vi "Main.vi"(8 "error in (no error)":errorcluster, 11 "Stop notifier":refnum<notifier>) -> (0 "error out":errorcluster)   [LabVIEW 2017, in "Temp.lvlib"]
doc: "Module main"
uses:
  Temp.lvlib
  ctl/StateData.ctl
  ctl/MainStates.ctl
  <vilib>/ErrorRing/Error Ring.xnode
  Error/Error.lvlib
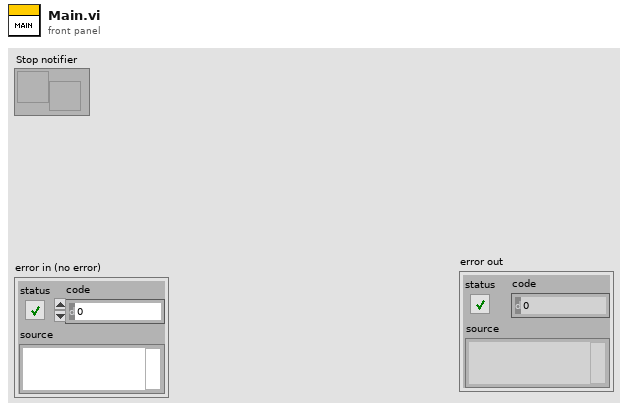
[diagram p1: front panel]
types:
  T1 = typedef "Temp.lvlib/StateData.ctl" = cluster{"Blank":dbl}
  T2 = typedef "Temp.lvlib/MainStates.ctl" = enum16{"Timeout", "Error", "Exit", "Init"}
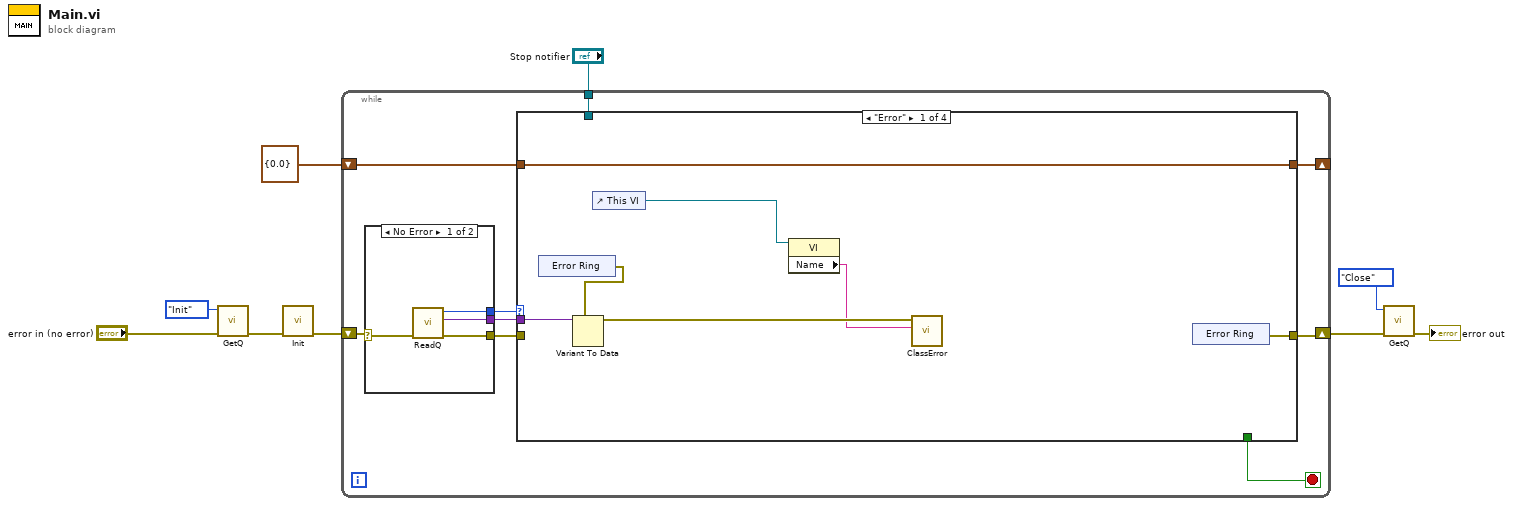
[diagram p0: block diagram]
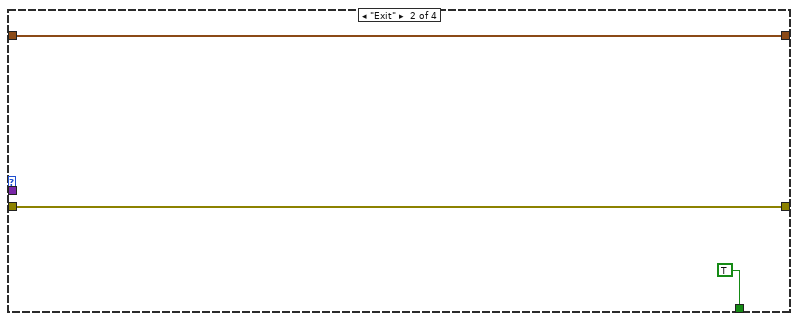
[diagram p2: hidden frame]
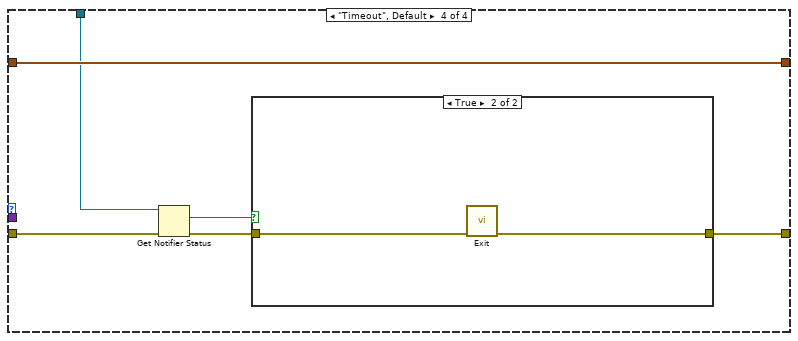
[diagram p4: hidden frame]
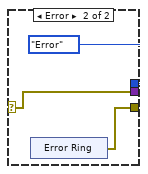
[diagram p6: hidden frame]
diagram:
  n1 = call "GetQ.vi"("error in (no error)"="error in (no error)", "Mode (Get)"=enum16{"Get", "Close", "Init"}."Init") -> ("error out"=w2:errorcluster)  [unwired: 8 in, 1 out]
  n2 = call "Init.vi"("error in (no error)"=w2) -> ("error out"=w1:errorcluster)  [unwired: 10 in]
  n3 = while {
    shift-right: [w14] -> w6
    shift-left: w1 -> [w18]
    shift-right: [w11] -> _
    shift-left: T1 {"Blank"=0.0} ("Cluster") -> [w12]
    tunnel: "Stop notifier" -> [w10]
    stop <- w13 stop-if-true
    n4 = case shown="No Error" w18 {
      selector: w18 -> [w45 w47]
      tunnel: [w44 MainStates."Error" ("State")] -> w17
      tunnel: [w43 w47] -> w16
      tunnel: [w42 w46] -> w15
      frame No Error {
        n5 = call "ReadQ.vi"("error in (no error)"=w45) -> ("error out"=w42:errorcluster, "Variant"=w43:variant, "State"=w44:T2)  [unwired: 8 in]
      }
      frame Error {
        n6 = xnode "Error Ring"() -> ("error out"=w46:errorcluster)
      }
    }
    n7 = case shown="\"Error\"" w17 {
      tunnel: w16 -> [w25 _ _ _]
      tunnel: w15 -> [_ w30 w32 w37]
      tunnel: [w24 w30 w32 w34] -> w14
      tunnel: [_ TRUE _ _] -> w13
      tunnel: w12 -> [w22 w28 w31 w38]
      tunnel: [w22 w28 w31 w38] -> w11
      tunnel: w10 -> [_ _ _ w36]
      frame "Error" {
        n8 = xnode "Error Ring"() -> ("error out"=w23:errorcluster)
        n9 = Variant To Data(type=w23, Variant=w25) -> (data=w21:errorcluster)  [unwired: 1 in, 1 out]
        n10 = control-ref of="This VI"() -> (w20:refnum<vi>)
        n11 = property class="VI"(reference=w20) -> ("Name"=w19:string)  [unwired: 1 in, 2 out]
        n12 = call "ClassError.vi"("From"=w19, "error in"=w21) -> ()  [unwired: 9 in, 1 out]
        n13 = xnode "Error Ring"() -> ("error out"=w24:errorcluster)
      }
      frame "Exit" {
      }
      frame "Init" {
      }
      frame "Timeout", Default {
        n14 = Get Notifier Status(notifier=w36, error in (no error)=w37) -> (current notification=w35:bool, error out=w33:errorcluster)  [unwired: 3 out]
        n15 = case shown="True" w35 {
          tunnel: [w39 w40] -> w34
          tunnel: w33 -> [w39 w41]
          frame False {
          }
          frame True {
            n16 = call "Exit.vi"("error in (no error)"=w41) -> ("error out"=w40:errorcluster)  [unwired: 10 in]
          }
        }
      }
    }
  }
  n17 = call "GetQ.vi"("error in (no error)"=w6, "Mode (Get)"=enum16{"Get", "Close", "Init"}."Close") -> ("error out"=→"error out":errorcluster)  [unwired: 8 in, 1 out]
